vi "Globalt0.vi"() -> ()   [LabVIEW 2022 SP3]
panel:
  in  "current time":timestamp
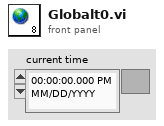
[diagram p1: front panel]
diagram:
